vi "SetAutoscaleOff.vi"(11 "Graph Reference Cluster":T1) -> ()   [LabVIEW 2014]
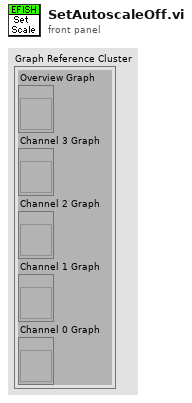
[diagram p1: front panel]
types:
  T1 = cluster{"Overview Graph":refnum<vi>, "Channel 3 Graph":refnum<vi>, "Channel 2 Graph":refnum<vi>, "Channel 1 Graph":refnum<vi>, "Channel 0 Graph":refnum<vi>}
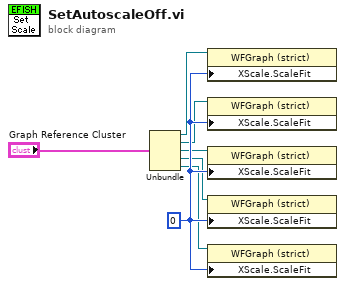
[diagram p0: block diagram]
diagram:
  w7 = u8 0 ("X Scale.Scale Fit")
  n1 = Unbundle("Graph Reference Cluster") -> ("Overview Graph"=w5:refnum<vi>, "Channel 3 Graph"=w4:refnum<vi>, "Channel 2 Graph"=w3:refnum<vi>, "Channel 1 Graph"=w2:refnum<vi>, "Channel 0 Graph"=w1:refnum<vi>)
  n2 = property on="Property Node" class="WFGraph (strict)"(reference=w5, "XScale.ScaleFit"=w7) -> ()  [unwired: 1 in, 2 out]
  n3 = property on="Property Node" class="WFGraph (strict)"(reference=w4, "XScale.ScaleFit"=w7) -> ()  [unwired: 1 in, 2 out]
  n4 = property on="Property Node" class="WFGraph (strict)"(reference=w3, "XScale.ScaleFit"=w7) -> ()  [unwired: 1 in, 2 out]
  n5 = property on="Property Node" class="WFGraph (strict)"(reference=w2, "XScale.ScaleFit"=w7) -> ()  [unwired: 1 in, 2 out]
  n6 = property on="Property Node" class="WFGraph (strict)"(reference=w1, "XScale.ScaleFit"=w7) -> ()  [unwired: 1 in, 2 out]
